vi "GEvt-Generate Complete Log.vi"(0 "CSM Global Log Event":T4, 2 "Event Data":T1={"Name (\"\" to Use UUID)"="", "Current State"="", "Arguments"="", "Source Message"={"‘State"="", "’Arguments"="", "’Error"={"status"=FALSE, "code"=0, "source"=""}}, "Source Module"="", "Complete(T)/Start(F)"=FALSE, "LogType"=enum."State Change", "Time Stamp"=timestamp(0 s since 1904-01-01)}, 5 "Error in":errorcluster caption="Error in (no error)", 7 "Enable?":bool=TRUE, 10 "CSM:LogFilter.lvclass":refnum<class "LogFilter.lvclass">) -> (14 "CSM Global Log Event Out":T4, 19 "Error out":errorcluster)   [LabVIEW 2017, in "Communicable State Machine.lvlib"]
doc: "### GEvt-Generate Complete Log.vi\n\n-- <b>Controls</b> --\n- <b>CSM Global Log Event</b>:\n- <b>event data</b>:\n- <b>Enable?</b>:\n- <b>CSM:LogFilter.lvclass</b>:\n\n-- <b>Indicators</b> --\n- <b>CSM Global Log Event out</b>:"
uses:
  Communicable State Machine.lvlib
  GEvt-Refs.ctl
  Typedef/_CSM_GlobalLog_MSG.ctl
  Typedef/_CSM_Response Source Message.ctl
  Typedef/_CSM_GlobalLog_MSG_TYPE.ctl
  LogFilter/LogFilter.lvclass
  LogFilter/LogFilter - Check.vi
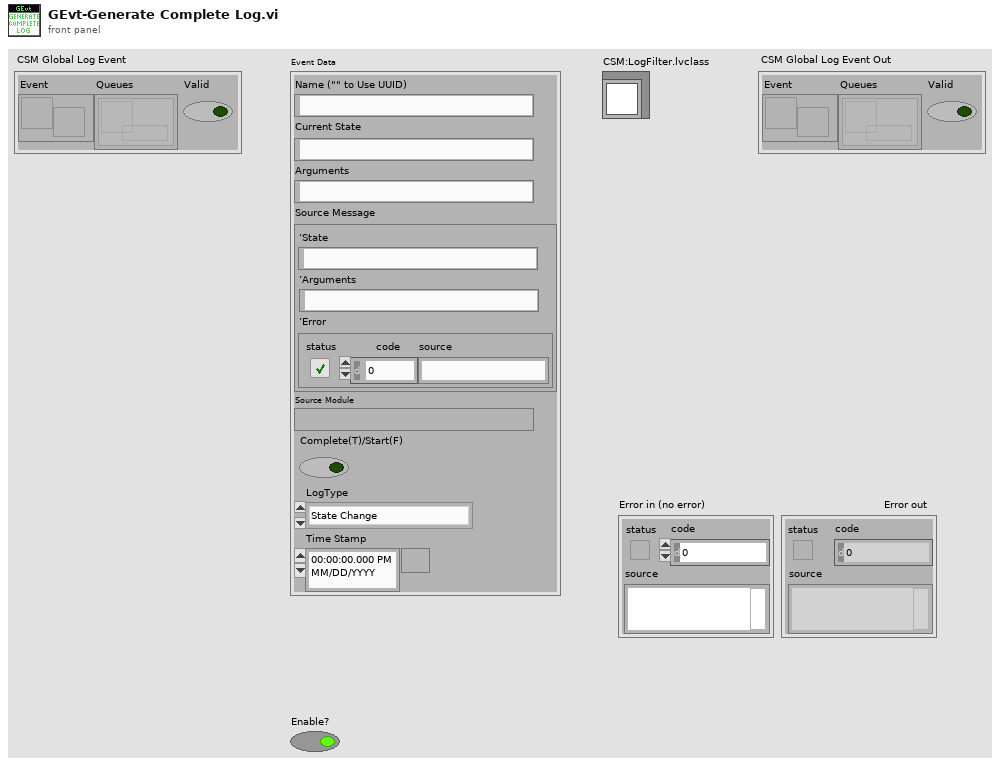
[diagram p1: front panel]
types:
  T1 = typedef "Communicable State Machine.lvlib/_CSM_GlobalLog_MSG.ctl" = cluster{"Name (\"\" to Use UUID)":string, "Current State":string, "Arguments":string, "Source Message":T2, "Source Module":string, "Complete(T)/Start(F)":bool, "LogType":T3, "Time Stamp":timestamp}
  T2 = typedef "Communicable State Machine.lvlib/_CSM_Response Source Message.ctl" = cluster{"‘State":string, "’Arguments":string, "’Error":errorcluster}
  T3 = typedef "Communicable State Machine.lvlib/_CSM_GlobalLog_MSG_TYPE.ctl" = enum16{"User Log", "State Change", "Status", "Interrupt", "Register", "Unregister", "Error Log", "Module Created", "Module Destroyed", "Async Message", "No-Rep Async Message", "Sync Message", "Async Message Complete", "Sync Message Complete"}
  T4 = typedef "Communicable State Machine.lvlib/GEvt-Refs.ctl" = cluster{"Event":refnum<user-event>, "Queues":refnum<queue>[], "Valid":bool}
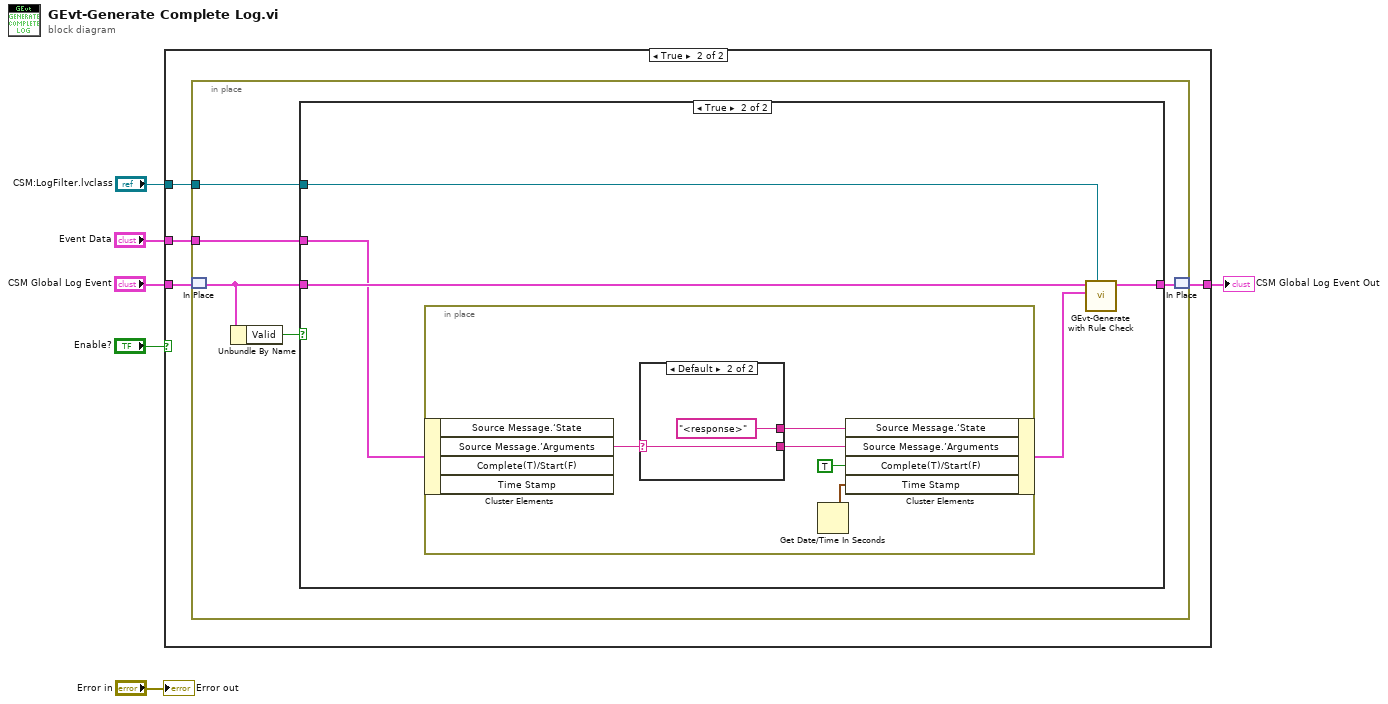
[diagram p0: block diagram]
diagram:
  n1 = case shown="True" "Enable?" {
    tunnel: "CSM Global Log Event" -> [w7 w11]
    tunnel: [w7 w10] -> w5
    tunnel: "Event Data" -> [_ w9]
    tunnel: "CSM:LogFilter.lvclass" -> [_ w8]
    frame False {
    }
    frame True {
      n2 = in-place {
        in-place-border: w9 -> [w15]
        in-place-border: w8 -> [w14]
        n3 = in-place-match #1(w11) -> (w13:T4)
        n4 = Unbundle By Name(w13) -> ("Valid"=w12:bool)
        n5 = case shown="True" w12 {
          tunnel: w13 -> [w17 w22]
          tunnel: [w17 w21] -> w16
          tunnel: w15 -> [_ w19]
          tunnel: w14 -> [_ w20]
          frame False {
          }
          frame True {
            n6 = in-place {
              n7 = in-place-cluster #2(w19) -> ("Source Message.’Arguments"=w26:string)  [unwired: 3 out]
              n8 = case shown="Default" w26 {
                selector: w26 -> [_ w28]
                tunnel: [_ "<response>" ("Source Message.‘State")] -> w27
                tunnel: [_ w28] -> w25
                frame "" {
                }
                frame Default {
                }
              }
              n9 = Get Date/Time In Seconds() -> (seconds since 1Jan1904=w23:timestamp)
              n10 = in-place-cluster #2("Source Message.‘State"=w27, "Source Message.’Arguments"=w25, "Complete(T)/Start(F)"=TRUE, "Time Stamp"=w23) -> (w18:T1)
            }
            n11 = call "GEvt-Generate with Rule Check.vi"("LogFilter In"=w20, "Event Data"=w18, "CSM Global Log Event In"=w22) -> ("CSM Global Log Event Out"=w21:T4)  [unwired: 8 in]
          }
        }
        n12 = in-place-match #1(w16) -> (w10:T4)
      }
    }
  }
  "CSM Global Log Event Out" <- w5
  "Error out" <- "Error in"
